vi "configure.vi"(8 "error in (no error)":errorcluster, 11 "SegmenterDL100224ThreeD in":refnum<class "SegmenterDL100224ThreeD.lvclass">) -> (0 "error out":errorcluster, 3 "SegmenterDL100224ThreeD out":refnum<class "SegmenterDL100224ThreeD.lvclass">)   [LabVIEW 2010, in "SegmenterDL100224ThreeD.lvclass"]
doc: "The dynamic dispatch version of this VI loads and displays the configuration file associated with the plug-in object. The user modify and save the configuration data."
uses:
  SegmenterDL100224ThreeD.lvclass
  SegmenterDL100224ThreeD.lvclass/SegmenterDL100224ThreeD.ctl
  common/classes/GenericComponent/GenericComponent/GenericComponent.lvclass
panel:
  in  "Preprocessing macro path":path
  in  "cancel button":bool
  in  "save button":bool
  out "Configuration":string
  # "Configure SegmenterDL100224ThreeD"
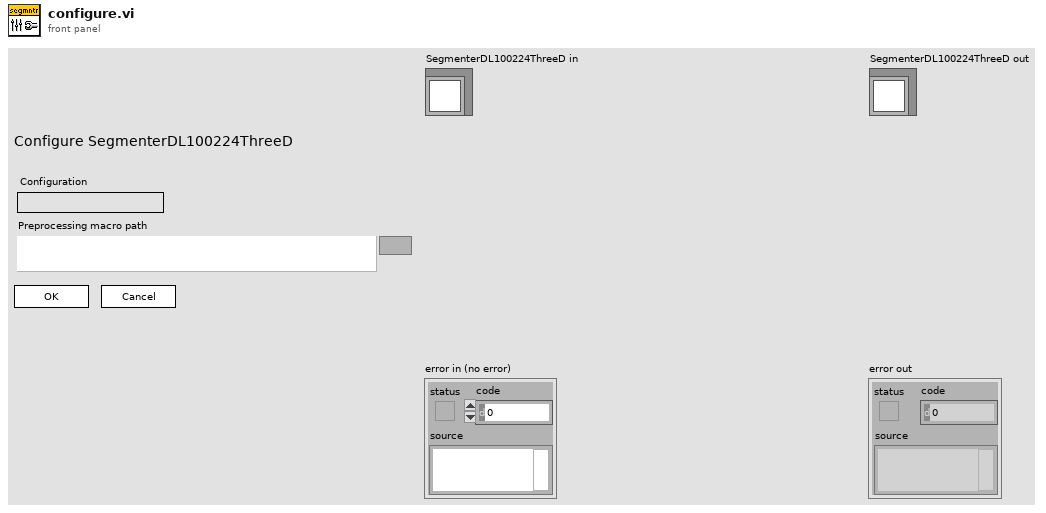
[diagram p1: front panel]
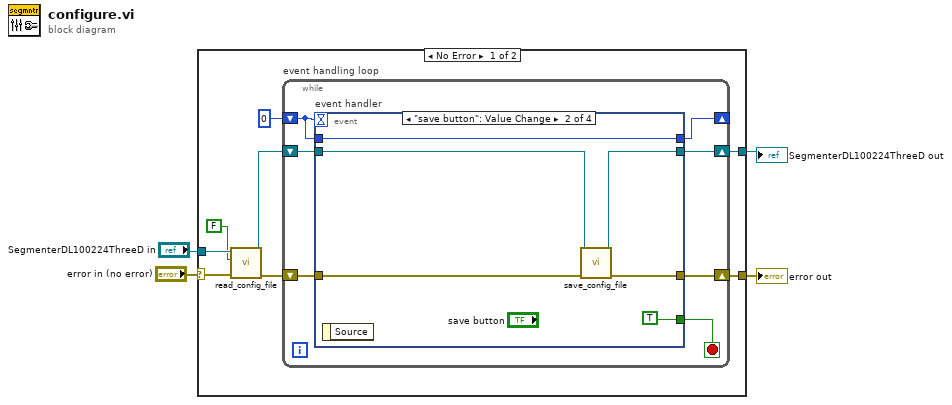
[diagram p0: block diagram]
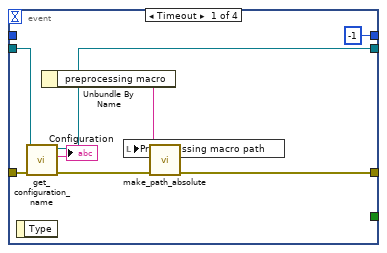
[diagram p2: hidden frame]
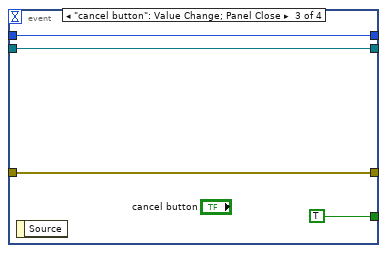
[diagram p3: hidden frame]
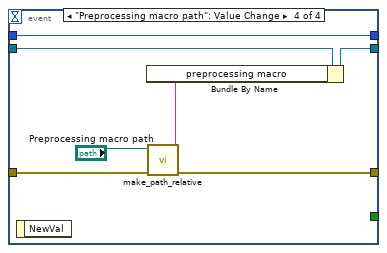
[diagram p4: hidden frame]
diagram:
  n1 = case shown="No Error" "error in (no error)" {
    selector: "error in (no error)" -> [w12 w47]
    tunnel: [w10 w47] -> w4
    tunnel: "SegmenterDL100224ThreeD in" -> [w9 w46]
    tunnel: [w5 w46] -> w3
    frame No Error {
      n2 = call-dynamic "read_config_file.vi"("error in (no error)"=w12, "force load?"=FALSE, "GenericPlugin in"=w9) -> ("error out"=w11:errorcluster, "GenericPlugin out"=w7:refnum<class "SegmenterDL100224ThreeD.lvclass">)  [unwired: 7 out]
      n3 = while "event handling loop" {
        shift-right: [w18] -> w10
        shift-left: w11 -> [w19]
        shift-right: [w15] -> w5
        shift-left: w7 -> [w17]
        shift-right: [w14] -> _
        shift-left: 0 -> [w16]
        stop <- w13 stop-if-true
        n4 = event "event handler" shown="[1] \"save button\": Value Change" {
          selector: _ -> [_ _ _ _]
          dyn-events: _ -> [_ _ _ _]
          timeout: w16 -> [_ _ _ _]
          tunnel: w19 -> [w27 w33 w38 w41]
          tunnel: [w22 w32 w38 w40] -> w18
          tunnel: w17 -> [w26 w29 w36 w44]
          tunnel: w16 -> [_ w34 w37 w45]
          tunnel: [-1 w34 w37 w45] -> w14
          tunnel: [w25 w31 w36 w43] -> w15
          tunnel: [_ TRUE TRUE _] -> w13
          event Timeout {
            n5 = event-data() -> ()  [unwired: 2 out]
            n6 = call "get_configuration_name.vi"("error in (no error)"=w27, "GenericPlugin.lvclass in"=w26) -> ("error out"=w23:errorcluster, "configuration name"=→"Configuration":string, "GenericPlugin.lvclass out"=w25:refnum<class "SegmenterDL100224ThreeD.lvclass">)  [unwired: 7 in]
            n7 = Unbundle By Name(w25) -> ("preprocessing macro"=w21:string)
            n8 = call "make_path_absolute.vi"("error in (no error)"=w23, "relative path"=w21) -> ("error out"=w22:errorcluster, "absolute path"=w20:path)  [unwired: 8 in]
            n9 = local write "Preprocessing macro path"(w20) -> ()
          }
          event "save button": Value Change {
            n10 = event-data() -> ()  [unwired: 2 out]
            n11 = call-dynamic "save_config_file.vi"("error in (no error)"=w33, "GenericPlugin in"=w29) -> ("error out"=w32:errorcluster, "GenericPlugin out"=w31:refnum<class "SegmenterDL100224ThreeD.lvclass">)  [unwired: 1 in, 7 out]
          }
          event "cancel button": Value Change; Panel Close {
            n12 = event-data() -> ()  [unwired: 2 out]
          }
          event "Preprocessing macro path": Value Change {
            n13 = event-data() -> ()  [unwired: 2 out]
            n14 = call "make_path_relative.vi"("error in (no error)"=w41, "absolute path"="Preprocessing macro path") -> ("error out"=w40:errorcluster, "relative path"=w39:string)  [unwired: 8 in]
            n15 = Bundle By Name(cluster=w44, "preprocessing macro"=w39) -> (w43:refnum<class "SegmenterDL100224ThreeD.lvclass">)
          }
        }
      }
    }
    frame Error {
    }
  }
  "error out" <- w4
  "SegmenterDL100224ThreeD out" <- w3
